vi "Unflatten.vi"(8 "error in (no error)":errorcluster, 9 "Timeout":bool, 10 "DAQ In":T1[](array[typedef]), 11 "CIF_NIChn_FIFO_DAQ in":refnum<class "CIF_NIChn_FIFO_DAQ.lvclass">) -> (0 "error out":errorcluster, 1 "Header":T2, 2 "DAQ Out":T1[](array[typedef]), 3 "CIF_NIChn_FIFO_DAQ out":refnum<class "CIF_NIChn_FIFO_DAQ.lvclass">)   [LabVIEW 2021, in "CIF_NIChn_FIFO_DAQ.lvclass"]
uses:
  CIF_NIChn_FIFO_DAQ.lvclass
  D:/dev/Packages/Channel_Manager/src/CIFChannels/CIFChannels.lvclass
  D:/dev/Packages/Channel_Manager/src/CIF_NIChn/FIFO_U8/CIF_NIChn_Fifo_U8.lvclass
  ChannelCommon/typedef/FIFO Header.ctl
  ChannelCommon/typedef/Datatype Waveform.ctl
  CIFChannels/CIFChannels.lvclass/CIFChannels.ctl
  FIFO_U8/CIF_NIChn_Fifo_U8.lvclass/CIF_NIChn_Fifo_U8.ctl
  <vilib>/CIF Foundation/CIF Utilities/Statistics/I64/Stats_I64_CIF_U.lvclass/Stats_I64_CIF_U.ctl
  4ab41953-a001-49d2-beab-55370b6c3c42.vi
  7cd889b7-face-4678-a9e3-2692853b6930.vi
  FIFO_U8/Accessors/Read Payload.vi
  FIFO_U8/Accessors/Write Payload.vi
  CIFChannels/Accessors/Write FIFO Timeout.vi
  <vilib>/CIF Foundation/CIF Utilities/Time/System Time/Get System Time.vi
  <vilib>/CIF Foundation/CIF Utilities/Statistics/I64/X1 minus X0.vi
  ChannelCommon/Utilities/Unflatten Header.vi
  <vilib>/CIF Foundation/CIF Utilities/DataTypes/Unflatten I64.vi
  ChannelCommon/CIFFIFO/Flatten/Waveform Unflatten.vi/ce8ba92d-590f-4e46-8b1c-68dfd5c82777.vi
  ChannelCommon/CIFFIFO/Flatten/Waveform Unflatten.vi/8980f996-a542-42f1-9c98-910966e77ad2.vi
  <vilib>/CIF Foundation/CIF Utilities/DataTypes/Unflatten U64.vi
  <vilib>/CIF Foundation/CIF Utilities/Time/System Time/LabVIEW Time to TAI Time.vi
  <vilib>/CIF Foundation/CIF Utilities/Statistics/I64/X1 minus X0.vi/dfabcf33-0dbc-4041-80a5-3dc0c86d2989.vi
  ChannelCommon/Utilities/Add Error.vi
  ChannelCommon/CIFFIFO/Flatten/Waveform Unflatten.vi/ce8ba92d-590f-4e46-8b1c-68dfd5c82777.vi/c28b0ead-42ad-4072-80a2-aca7f2bd7ce3.vi
  ChannelCommon/CIFFIFO/Flatten/Waveform Unflatten.vi/8980f996-a542-42f1-9c98-910966e77ad2.vi/c28b0ead-42ad-4072-80a2-aca7f2bd7ce3.vi
  <vilib>/CIF Foundation/CIF Utilities/Statistics/I64/X1 minus X0.vi/dfabcf33-0dbc-4041-80a5-3dc0c86d2989.vi/9eb60a9a-770f-4d2d-8b3f-8465c267ecc9.vi
  <vilib>/CIF Foundation/CIF Utilities/Errors/Append Error Location.vi
  CIFChannels/CIFChannels.lvclass
  ChannelCommon/ChannelCommon.lvlib
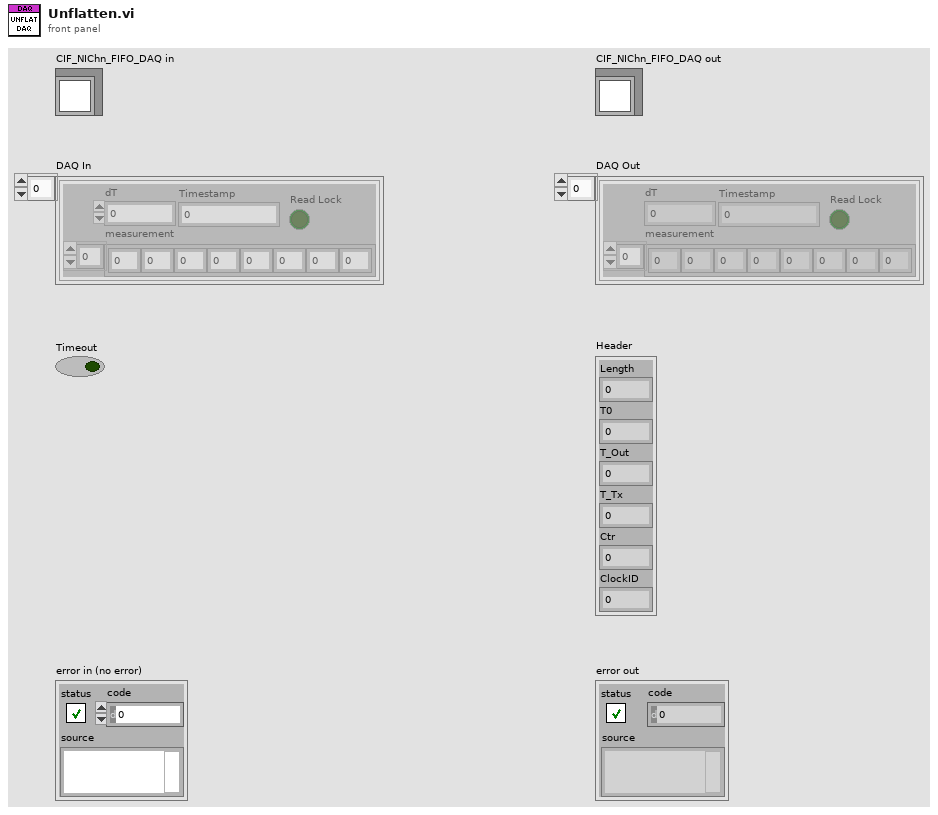
[diagram p1: front panel]
types:
  T1 = typedef "ChannelCommon.lvlib/Datatype Waveform.ctl" = cluster{"measurement":dbl[], "dT":dbl, "Timestamp":i64, "Read Lock":bool}
  T2 = typedef "ChannelCommon.lvlib/FIFO Header.ctl" = cluster{"Length":u64, "T0":i64, "T_Out":i64, "T_Tx":i64, "Ctr":u64, "ClockID":u8}
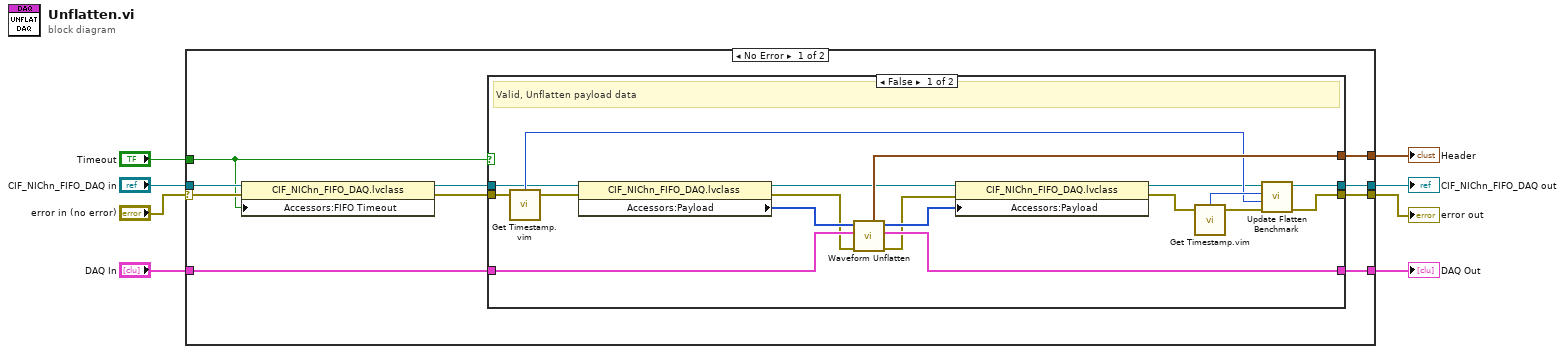
[diagram p0: block diagram]
diagram:
  n1 = case shown="No Error" "error in (no error)" {
    selector: "error in (no error)" -> [w13 w42]
    tunnel: [w16 w42] -> w5
    tunnel: [w17 w41] -> w6
    tunnel: "CIF_NIChn_FIFO_DAQ in" -> [w12 w41]
    tunnel: [w18 _] -> w7
    tunnel: "Timeout" -> [w11 _]
    tunnel: "DAQ In" -> [w10 w40]
    tunnel: [w9 w40] -> w8
    frame No Error {
      n2 = property class="CIF_NIChn_FIFO_DAQ.lvclass"(reference=w12, error in=w13, "Accessors:FIFO Timeout"=w11) -> (reference out=w15:refnum<class "CIF_NIChn_FIFO_DAQ.lvclass">, error out=w14:errorcluster)
      n3 = case shown="False" w11 {
        tunnel: w14 -> [w36 w38]
        tunnel: w15 -> [w27 w39]
        tunnel: [w31 _] -> w18
        tunnel: [w35 w39] -> w17
        tunnel: [w34 w38] -> w16
        tunnel: w10 -> [w33 w37]
        tunnel: [w32 w37] -> w9
        frame False {
          # "Valid, Unflatten payload data"
          n4 = call "Get Timestamp.vim"("Anything in"=w36) -> ("Time (ns)"=w29:i64, "Anything out"=w22:errorcluster)  [unwired: 2 in]
          n5 = property class="CIF_NIChn_FIFO_DAQ.lvclass"(reference=w27, error in=w22) -> (reference out=w25:refnum<class "CIF_NIChn_FIFO_DAQ.lvclass">, error out=w21:errorcluster, "Accessors:Payload"=w26:u8[])
          n6 = call "Waveform Unflatten.vi"("error in (no error)"=w21, "Data in in"=w33, "Flatten Data in"=w26) -> ("error out"=w20:errorcluster, "Data out"=w32:T1[], "Flatten Data out"=w24:u8[], "Header out"=w31:T2)  [unwired: 5 in]
          n7 = property class="CIF_NIChn_FIFO_DAQ.lvclass"(reference=w25, error in=w20, "Accessors:Payload"=w24) -> (reference out=w23:refnum<class "CIF_NIChn_FIFO_DAQ.lvclass">, error out=w19:errorcluster)
          n8 = call "Get Timestamp.vim"("Anything in"=w19) -> ("Time (ns)"=w30:i64, "Anything out"=w28:errorcluster)  [unwired: 2 in]
          n9 = call "Update Flatten Benchmark.vi"("error in (no error)"=w28, "X0"=w29, "X1"=w30, "CIFChannels in"=w23) -> ("error out"=w34:errorcluster, "CIFChannels out"=w35:refnum<class "CIF_NIChn_FIFO_DAQ.lvclass">)  [unwired: 6 in]
        }
        frame True {
          # "Timeout"
        }
      }
    }
    frame Error {
    }
  }
  "error out" <- w5
  "CIF_NIChn_FIFO_DAQ out" <- w6
  "Header" <- w7
  "DAQ Out" <- w8
